vi "Kinematic_Calculations.vi"(0 "Width (ft)":dbl, 2 "Length (ft)":dbl, 3 "Max_Wheel_Speed (rpm)":dbl, 4 "Wheel_Diamater (in)":dbl) -> ()   [LabVIEW 2018]
uses:
  Global_Variables/Kinematic_Globals.vi
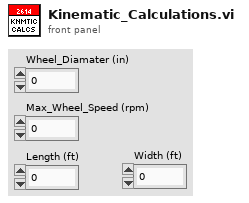
[diagram p1: front panel]
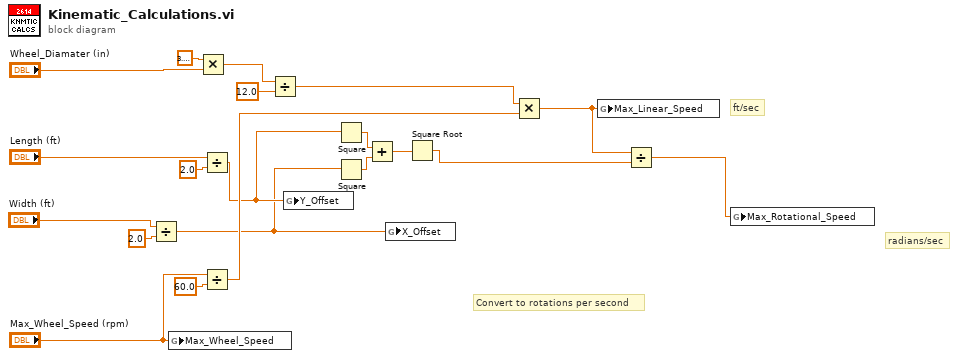
[diagram p0: block diagram]
diagram:
  # "ft/sec"
  # "radians/sec"
  # "Convert to rotations per second"
  n1 = Divide(x="Width (ft)", y=2.0) -> (x/y=w5:dbl)
  n2 = global write "Kinematic_Globals.vi" "Max_Wheel_Speed"("Max_Wheel_Speed (rpm)") -> ()
  n3 = Multiply(x=3.141592653589793, y="Wheel_Diamater (in)") -> (x*y=w4:dbl)
  n4 = Divide(x="Length (ft)", y=2.0) -> (x/y=w6:dbl)
  n5 = Divide(x="Max_Wheel_Speed (rpm)", y=60.0) -> (x/y=w16:dbl)
  n6 = Divide(x=w4, y=12.0) -> (x/y=w2:dbl)
  n7 = global write "Kinematic_Globals.vi" "Y_Offset"(w6) -> ()
  n8 = Square(x=w6) -> (x^2=w8:dbl)
  n9 = Square(x=w5) -> (x^2=w7:dbl)
  n10 = Add(x=w8, y=w7) -> (x+y=w9:dbl)
  n11 = global write "Kinematic_Globals.vi" "X_Offset"(w5) -> ()
  n12 = Square Root(x=w9) -> (sqrt(x)=w1:dbl)
  n13 = Multiply(x=w2, y=w16) -> (x*y=w15:dbl)
  n14 = global write "Kinematic_Globals.vi" "Max_Linear_Speed"(w15) -> ()
  n15 = Divide(x=w15, y=w1) -> (x/y=w14:dbl)
  n16 = global write "Kinematic_Globals.vi" "Max_Rotational_Speed"(w14) -> ()
